vi "Comparison Functions.vi"() -> ()   [LabVIEW 2023]
doc: "This example shows how the Equal? function operates with different data types. These concepts also apply to the Not Equal?, Greater?, Less?, Greater Or Equal?, Less Or Equal?, Equal To 0?, Not Equal To 0?, Greater Than 0?, Less Than 0?, Greater Or Equal To 0?, and Less Or Equal To 0? functions."
uses:
  <vilib>/Utility/traverseref.llb/TRef TravTarget.ctl
  <vilib>/Utility/traverseref.llb/VI Scripting - Traverse.lvlib
panel:
  in  "Tab Control":T1(tab)
  out "Numeric Result":bool
  in  "Numeric 2":i32=1
  in  "Numeric 1":i32=1
  out "String Result":bool
  in  "String 2":string="labview"
  in  "String 1":string="LabVIEW"
  out "Path Result":bool
  in  "Path 2":path=path "C:/TEST.TXT"
  in  "Path 1":path=path "c:/test.txt"
  out "Cluster Result":T2
  in  "Cluster 2":T3={"String"="test", "Numeric"=3.0, "Boolean"=TRUE}
  in  "Cluster 1":T3={"String"="test", "Numeric"=3.0, "Boolean"=TRUE}
  out "Numeric Refnum Value 2":u32
  out "Numeric Refnum Value 1":u32
  out "Refnum Result":bool
  in  "Time Stamp":timestamp
  out "Array to Scalar Result":bool[](array[boolean])
  in  "Scalar":dbl=2.0
  in  "Array":dbl[](array[numeric])=[1.0, 2.0, 3.0]
  out "Array to Array Result":bool[](array[boolean])
  in  "Array to Array 2":dbl[](array[numeric])=[1.0, 2.0, 3.0]
  in  "Array to Array 1":dbl[](array[numeric])=[1.0, 2.0, 3.0]
  # "Overview: Demonstrates how the Equal? function operates with different data types.\nInstructions:\n1. Run the VI.\n2. Examine the different cases.\n3. Although this example demonstrates the Equal? function, the concepts also apply to other Comparison functions, including all of the 'Greater' and 'Less' functions."
  # "Equal? will return TRUE if both numerics are the same value."
  # "Equal? will return TRUE if both strings are the same value. The comparison is case-sensitive, so 'LabVIEW' and 'labview' would not be considered equal."
  # "Equal? will return TRUE if both paths are the same value. The comparison is case-insensitive on some platforms (like Windows), and case-sensitive on other platforms (like Linux)."
  # "Equal? will return a cluster of Booleans with the same number of elements as the input clusters. Each Boolean will be TRUE if the corresponding elements in the clusters are the same value."
  # "Equal? will return TRUE if both refnums refer to the same control. This is the case, even if the refnums have different numeric values."
  # "Note: Control references from different sources are used for the refnum comparison. The actual value of this Time Stamp is not used in this example."
  # "When comparing arrays with arrays, Equal? will return an array of Booleans with the same number of elements as the smaller of the two input arrays. When comparing an array to a scalar, Equal? will return an array of Booleans with the same number of elements as the array."
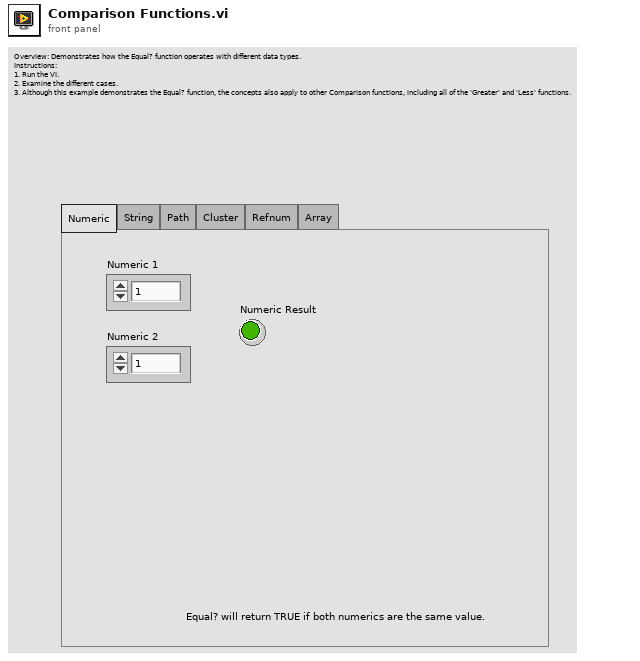
[diagram p1: front panel]
types:
  T1 = enum32{"Numeric", "String", "Path", "Cluster", "Refnum", "Array"}
  T2 = cluster{"String":bool, "Numeric":bool, "Boolean":bool}
  T3 = cluster{"String":string, "Numeric":dbl, "Boolean":bool}
  T4 = typedef "TRef TravTarget.ctl" = enum16{"FP", "BD", "Other"}
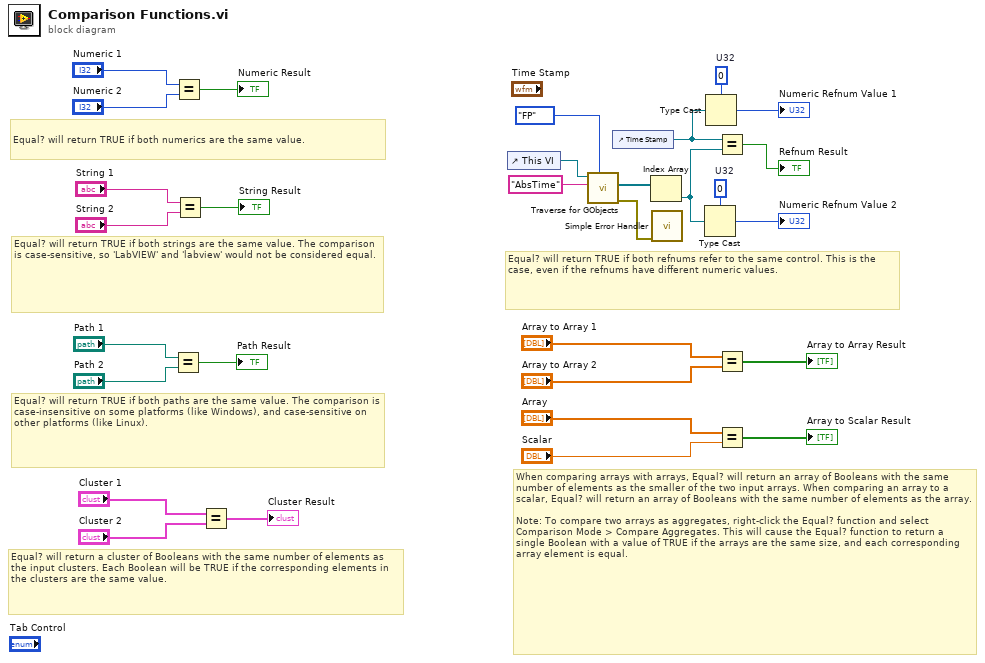
[diagram p0: block diagram]
diagram:
  w4 = u32 0  # U32
  w6 = u32 0  # U32
  # "When comparing arrays with arrays, Equal? will return an array of Booleans with the same number of elements as the smaller of the two input arrays. When comparing an array to a scalar, Equal? will return an array of Booleans with the same number of elements as the array.\n\nNote: To compare two arrays as aggregates, right-click the Equal? function and select Comparison Mode > Compare Aggregates. This will cause the Equal? function to return a single Boolean with a value of TRUE if the arrays are the same size, and each corresponding array element is equal."
  # "Equal? will return TRUE if both refnums refer to the same control. This is the case, even if the refnums have different numeric values."
  # "Equal? will return TRUE if both paths are the same value. The comparison is case-insensitive on some platforms (like Windows), and case-sensitive on other platforms (like Linux)."
  # "Equal? will return a cluster of Booleans with the same number of elements as the input clusters. Each Boolean will be TRUE if the corresponding elements in the clusters are the same value."
  # "Equal? will return TRUE if both strings are the same value. The comparison is case-sensitive, so 'LabVIEW' and 'labview' would not be considered equal."
  # "Equal? will return TRUE if both numerics are the same value."
  n1 = Equal?(x="Path 1", y="Path 2") -> (x = y?=→"Path Result":bool)
  n2 = Equal?(x="Numeric 1", y="Numeric 2") -> (x = y?=→"Numeric Result":bool)
  n3 = Equal?(x="String 1", y="String 2") -> (x = y?=→"String Result":bool)
  n4 = Equal?(x="Cluster 1", y="Cluster 2") -> (x = y?=→"Cluster Result":T2)
  n5 = control-ref of="This VI"() -> (w11:refnum<vi>)
  n6 = call <vilib>:"Traverse for GObjects.vi"("Traverse Target"=TRef_TravTarget."FP", "Class Name"="AbsTime", "VI Refnum"=w11) -> ("error out"=w8:errorcluster, "References"=w9:refnum<vi>[])  [unwired: 5 in, 2 out]
  n7 = control-ref of="Time Stamp"() -> (w3:refnum<vi>)
  n8 = Index Array(array=w9) -> (element=w7:refnum<vi>)  [unwired: 1 in]
  n9 = call <vilib>:"Simple Error Handler.vi"("error in (no error)"=w8) -> ()  [unwired: 4 in, 5 out]
  n10 = Type Cast(type=w6, x=w7) -> (*(type *) &x=→"Numeric Refnum Value 2":u32)
  n11 = Type Cast(type=w4, x=w3) -> (*(type *) &x=→"Numeric Refnum Value 1":u32)
  n12 = Equal?(x=w3, y=w7) -> (x = y?=→"Refnum Result":bool)
  n13 = Equal?(x="Array to Array 1", y="Array to Array 2") -> (x = y?=→"Array to Array Result":bool[])
  n14 = Equal?(x="Array", y="Scalar") -> (x = y?=→"Array to Scalar Result":bool[])
